vi "MasterSlavePattern 1.vi"() -> ()   [LabVIEW 2015]
doc: "Use this template to build a master/slave design pattern. The master loop always executes. It notifies one or more slave loops to execute their code. The slave loop(s) continue executing until they complete, then wait for another notification. Contrast this with the Producer/Consumer pattern in which the consumer loops execute only when they have data in their queue."
panel:
  in  "stop":bool
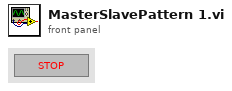
[diagram p1: front panel]
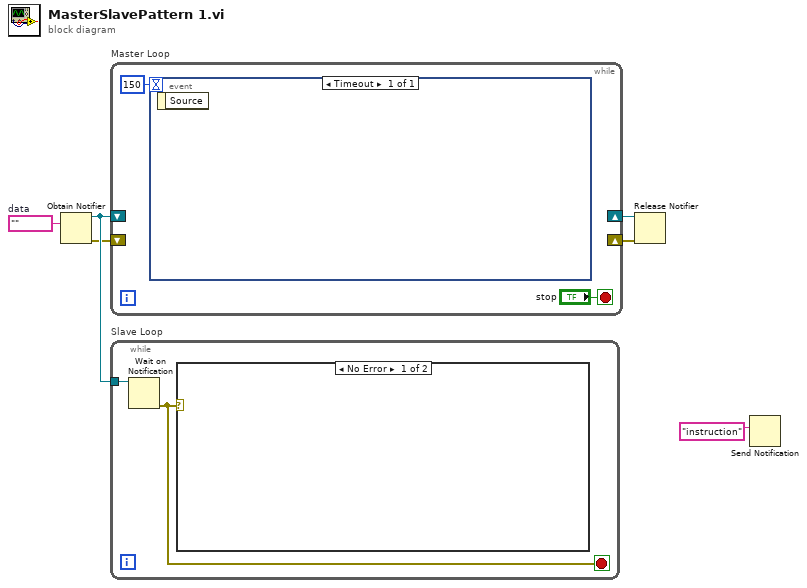
[diagram p0: block diagram]
diagram:
  w2 = ""  # data
  n1 = Obtain Notifier(notification data type=w2) -> (notifier out=w6:refnum<notifier>, error out=w5:errorcluster)  [unwired: 2 in, 2 out]
  n2 = while "Master Loop" {
    shift-right: [_] -> w4
    shift-left: w5 -> [_]
    shift-right: [_] -> w3
    shift-left: w6 -> [_]
    stop <- "stop" stop-if-true
    n3 = event shown="[0] Timeout" {
      selector: _ -> [_]
      dyn-events: _ -> [_]
      timeout: 150 -> [_]
      event Timeout {
        n4 = event-data() -> ()  [unwired: 1 in, 1 out]
      }
    }
  }
  n5 = while "Slave Loop" {
    tunnel: w6 -> [w10]
    stop <- w9 stop-if-true
    n6 = Wait on Notification(notifier=w10) -> (error out=w9:errorcluster)  [unwired: 1 in, 5 out]
    n7 = case shown="No Error" w9 {
      frame No Error {
      }
      frame Error {
      }
    }
  }
  n8 = Release Notifier(notifier=w3, error in (no error)=w4) -> ()  [unwired: 4 out]
  n9 = Send Notification(notification="instruction") -> ()  [unwired: 2 in, 2 out]
